vi "New Message Queue.vi"() -> (0 "error out":errorcluster, 3 "Message Queue out":refnum<class "Message Queue.lvclass">)   [LabVIEW 2019, in "Network Interface.lvlib" / "Message Queue.lvclass"]
uses:
  <vilib>/gpm_packages/@cs/Network-Sink/Source/Network Interface/Message Queue/Message Queue.lvclass
  <vilib>/gpm_packages/@cs/Network-Sink/Source/Network Interface/Message Queue/Message Cluster.ctl
  <vilib>/gpm_packages/@cs/Network-Sink/Source/Network Interface/Message Queue/Message Queue.lvclass/Message Queue.ctl
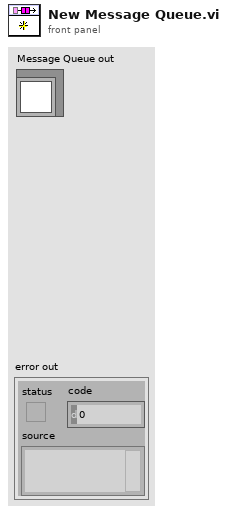
[diagram p1: front panel]
types:
  T1 = typedef "Network Interface.lvlib/Message Queue.lvclass/Message Cluster.ctl" = cluster{"Msg":string, "Data":variant}
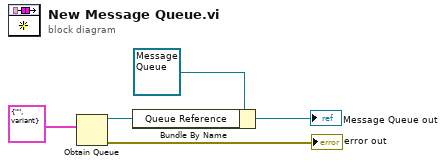
[diagram p0: block diagram]
diagram:
  n1 = Obtain Queue(element data type=T1 {"Msg"="", "Data"=variant} ("Cluster")) -> (queue out=w1:refnum<queue>, error out=→"error out":errorcluster)  [unwired: 4 in, 1 out]
  n2 = Bundle By Name(cluster=refnum<class "Message Queue.lvclass"> refnum ("Message Queue in"), "Queue Reference"=w1) -> (→"Message Queue out":refnum<class "Message Queue.lvclass">)
